vi "LabVIEW Data to Python String (I32).vi"(8 "error in (no error)":errorcluster, 10 "LabVIEW Data":i32) -> (0 "error out":errorcluster, 2 "Python String":string)   [LabVIEW 2020, in "jki_python_data_tools.lvlib"]
doc: "Writes a value associated with key in a specified section of the configuration data identified by refnum. If \"key\" input is not specified, the name of the variant object is used as the key.\n\nFor example a Boolean named \"Enable\" with a value of TRUE would correspond to the key-value pair:\n\nEnable=TRUE"
uses:
  jki_python_data_tools.lvlib
panel:
  # "Copyright © 2003-2009 JKI. All rights reserved.\n\nAuthor: Jim Kring [jim.kring@jameskring.com]\n\nThis library is provided \"AS IS\" ,WITHOUT WARRANTIES OR \nCONDITIONS OF ANY KIND, either express or implied.\n\nJames Kring, Inc. -- http://www.jameskring.com"
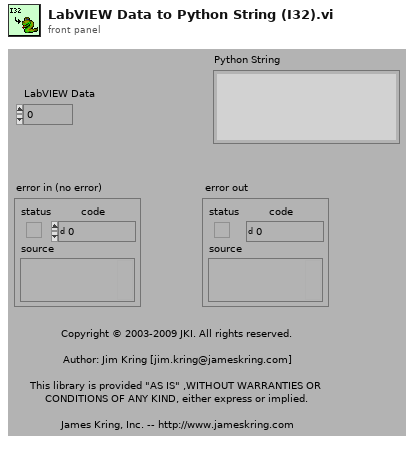
[diagram p1: front panel]
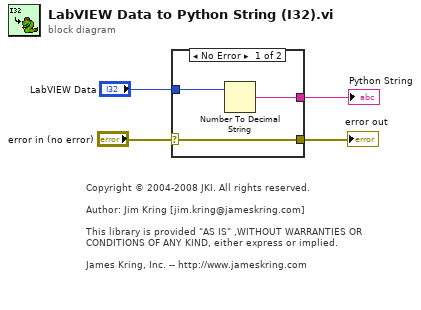
[diagram p0: block diagram]
diagram:
  # "Copyright © 2004-2008 JKI. All rights reserved.\n\nAuthor: Jim Kring [jim.kring@jameskring.com]\n\nThis library is provided \"AS IS\" ,WITHOUT WARRANTIES OR \nCONDITIONS OF ANY KIND, either express or implied.\n\nJames Kring, Inc. -- http://www.jameskring.com"
  n1 = case shown="No Error" "error in (no error)" {
    selector: "error in (no error)" -> [w5 w8]
    tunnel: "LabVIEW Data" -> [w7 _]
    tunnel: [w6 _] -> w1
    tunnel: [w5 w8] -> w4
    frame No Error {
      n2 = Number To Decimal String(number=w7) -> (decimal integer string=w6:string)  [unwired: 1 in]
    }
    frame Error {
    }
  }
  "error out" <- w4
  "Python String" <- w1
